vi "testUDPReciever.vi"() -> ()   [LabVIEW 2012]
panel:
  out "word 3":u8[](array[numeric]) format="%02x"
  out "word 2":u8[](array[numeric]) format="%02x"
  out "word 1":u8[](array[numeric]) format="%02x"
  out "word 0":u8[](array[numeric]) format="%02x"
  out "i":i32
  out "Found Header":bool
  out "MultiDimHeader":bool[][](array[boolean])
  out "NumBins":u32
  out "Cnts/Bin":u32
  out "Prof/Hist":u32
  out "Sync":u32
  out "Channel":u32
  out "rTime":u32
  out "frameCntr":u32
  out "subarray":bool[](array[boolean])
  out "channel 11":u32[](graph)
  out "in 11":bool
  out "channel 10":u32[](graph)
  out "in 10":bool
  out "channel 9":u32[](graph)
  out "in 9":bool
  out "channel 8":u32[](graph)
  out "in 8":bool
  out "channel 7":u32[](graph)
  out "in 7":bool
  out "channel 6":u32[](graph)
  out "in 6":bool
  out "channel 5":u32[](graph)
  out "in 5":bool
  out "channel 4":u32[](graph)
  out "in 4":bool
  out "channel 3":u32[](graph)
  out "in 3":bool
  out "channel 2":u32[](graph)
  out "in 2":bool
  out "channel 1":u32[](graph)
  out "in 1":bool
  out "channel 0":u32[](graph)
  out "in 0":bool
  out "appended array 2":string[](array[string])
  out "channel":u32
  out "appended array":bool[][](array[boolean])
  out "Found Header 2":bool
  out "word 7":u8[](array[numeric]) format="%02x"
  out "word 6":u8[](array[numeric]) format="%02x"
  out "word 5":u8[](array[numeric]) format="%02x"
  out "word 4":u8[](array[numeric]) format="%02x"
  out "Raw Data Out":string
  out "error post-check":errorcluster
  out "End Reciever Error":errorcluster
  in  "stop reciever":bool
  out "port":u16
  out "error out post-read":errorcluster
  out "error out pre-read":errorcluster
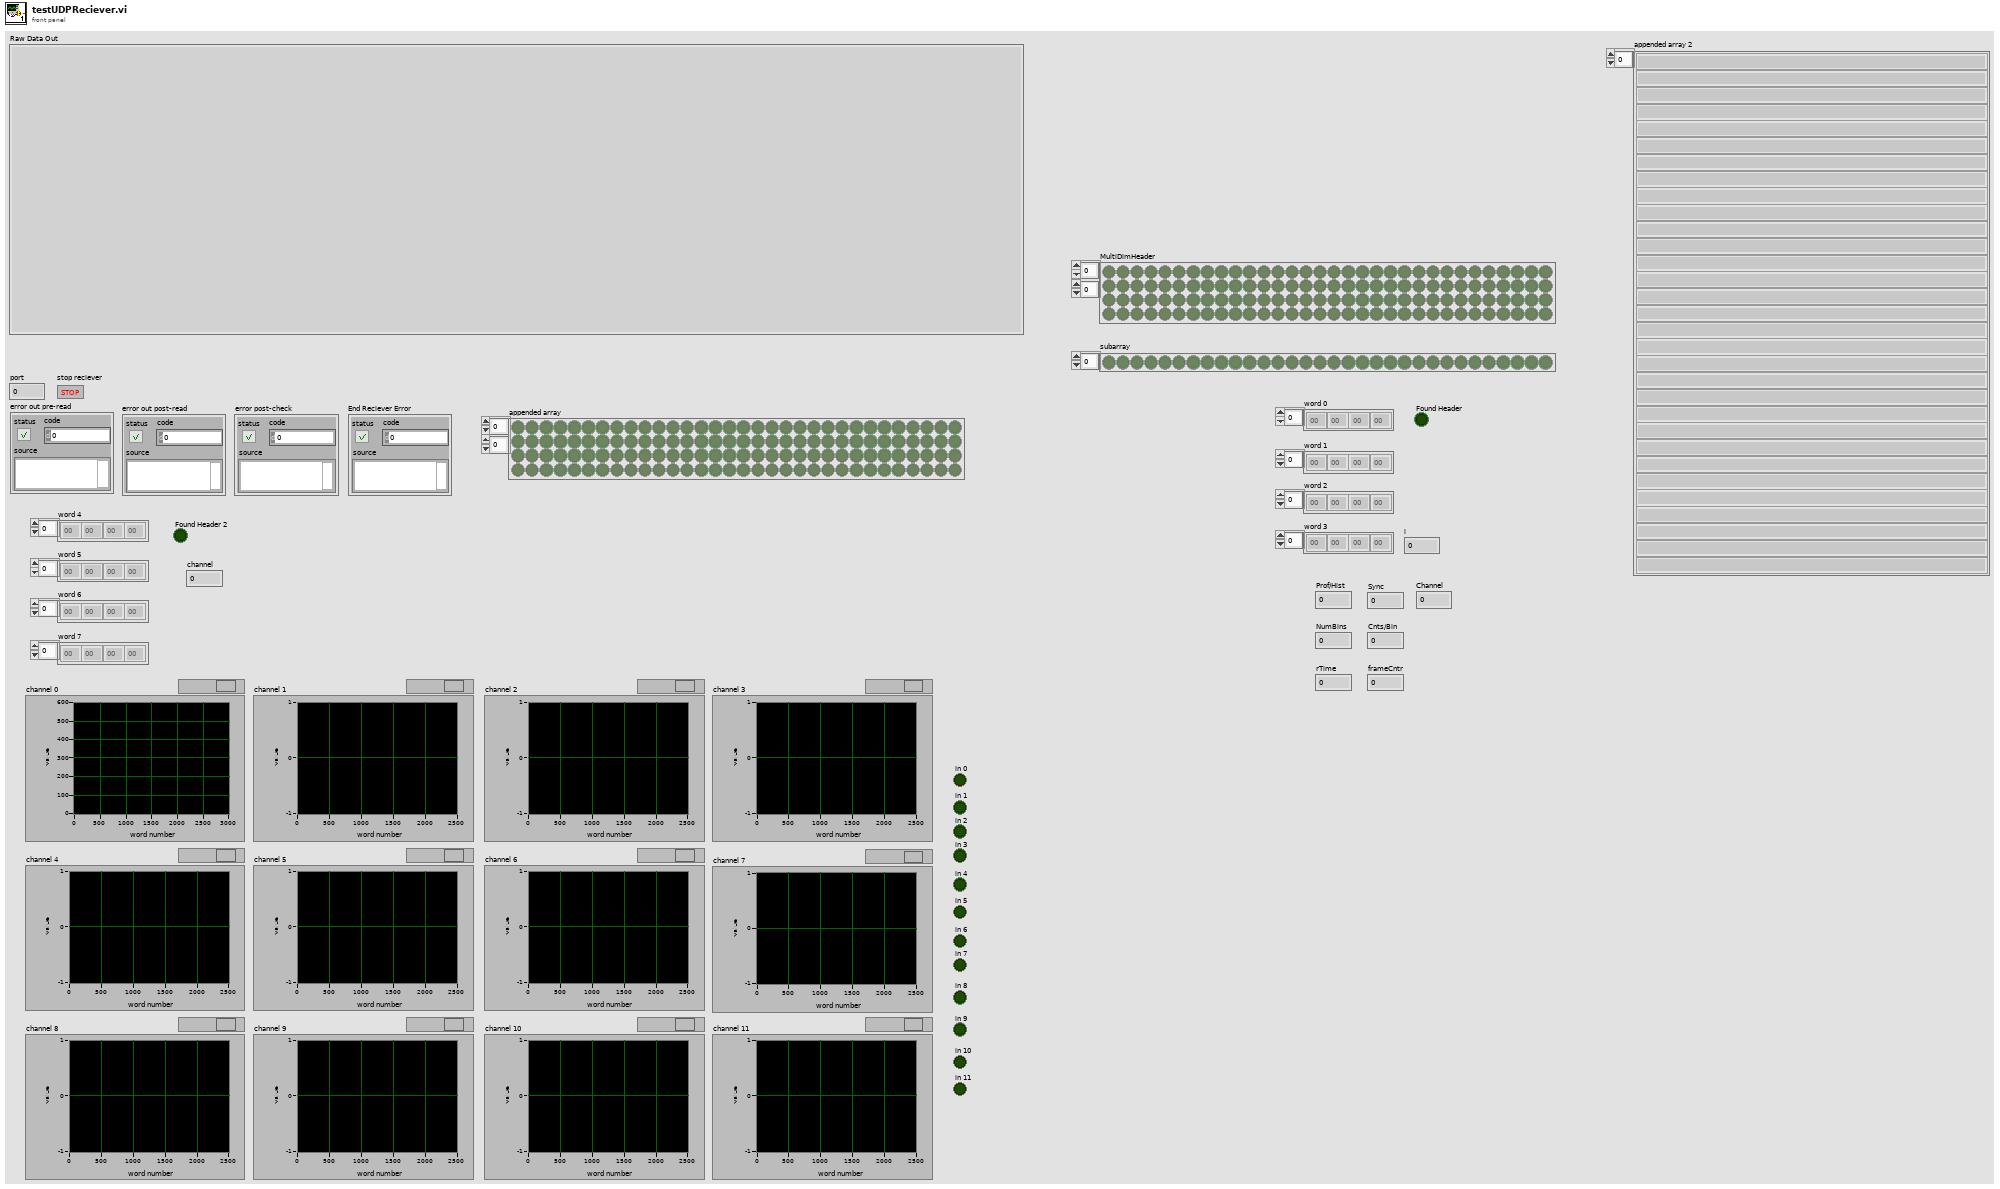
[diagram p1: front panel]
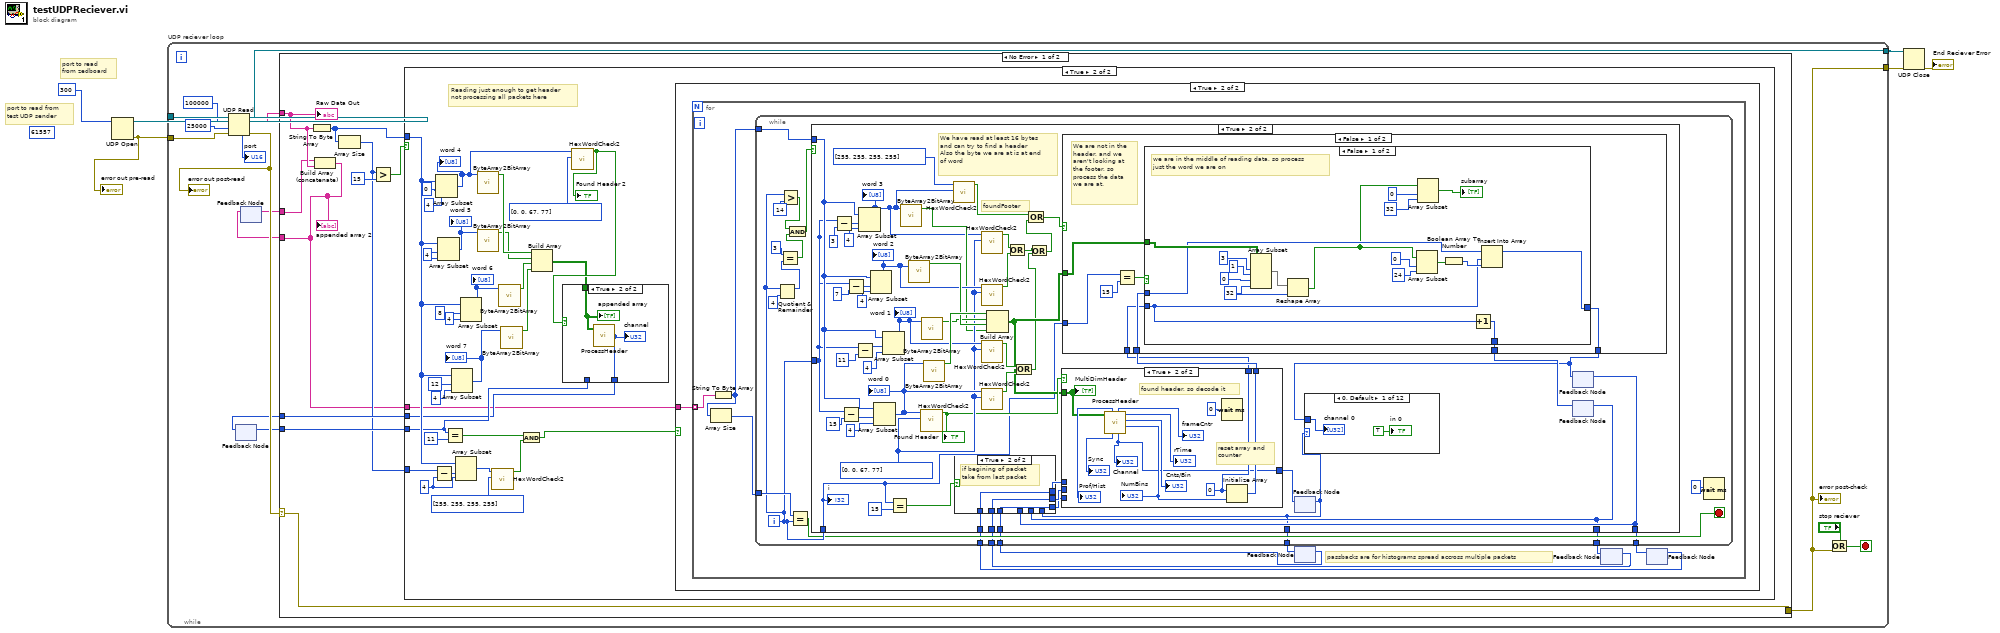
[diagram p0: block diagram]
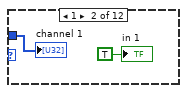
[diagram p5: hidden frame]
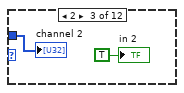
[diagram p6: hidden frame]
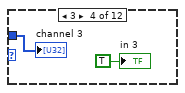
[diagram p7: hidden frame]
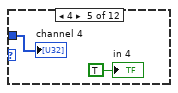
[diagram p8: hidden frame]
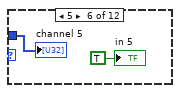
[diagram p9: hidden frame]
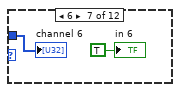
[diagram p10: hidden frame]
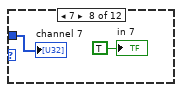
[diagram p11: hidden frame]
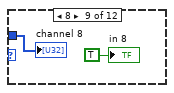
[diagram p12: hidden frame]
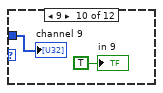
[diagram p13: hidden frame]
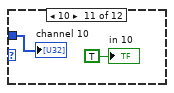
[diagram p14: hidden frame]
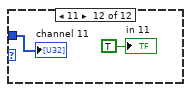
[diagram p15: hidden frame]
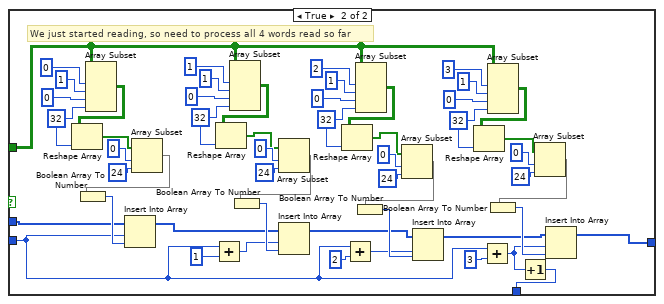
[diagram p17: hidden frame]
diagram:
  (unwired) u16 61557 ("port")
  # "port to read \nfrom zedboard"
  # "port to read from \ntest UDP sender"
  n1 = UDP Open(11:u16 300 ("port")) -> (port=w5:refnum<k16>, 0:w2:errorcluster)  [unwired: 4 in, 1 out]
  "error out pre-read" <- w2
  n2 = while "UDP reciever loop" {
    tunnel: [w21] -> w6
    tunnel: w5 -> [w20]
    tunnel: [w12] -> w4
    tunnel: w2 -> [w17]
    stop <- w19 stop-if-true
    n3 = UDP Read(connection ID=w20, max size (548)=100000, timeout ms (25000)=25000, 8:w17) -> (data out=w14:string, error out=w16:errorcluster, 3:w21:refnum<k16>, 4:→"port":u16)  [unwired: 1 out]
    "error out post-read" <- w16
    n4 = feedback #1() -> (w7:u32)  [unwired: 1 in]
    n5 = feedback #2() -> (w9:string[])  [unwired: 1 in]
    n6 = case shown="No Error" w16 {
      selector: w16 -> [w31 w278]
      tunnel: w14 -> [w30 _]
      tunnel: [w31 w278] -> w12
      tunnel: [w23 w277] -> w10
      tunnel: w9 -> [w29 w277]
      tunnel: [w26 w276] -> w8
      tunnel: w7 -> [w25 w276]
      frame No Error {
        n7 = String To Byte Array(string=w30) -> (unsigned byte array=w22:u8[])
        n8 = Build Array (concatenate)(w29, w30) -> (w23:string[])
        "appended array 2" <- w23
        n9 = Array Size(array=w22) -> (size(s)=w24:i32)
        n10 = Greater?(x=w24, y=15) -> (0:w28:bool)
        n11 = case shown="True" w28 {
          tunnel: w22 -> [_ w40]
          tunnel: [w32 w34] -> w26
          tunnel: w25 -> [w32 w35]
          tunnel: w24 -> [_ w37]
          tunnel: w23 -> [_ w33]
          frame False {
          }
          frame True {
            w39 = 4 ("length")
            w58 = 4 ("length")
            # "Reading just enough to get header\nnot processing all packets here"
            n12 = Subtract(x=w37, y=w39) -> (x-y=w38:i32)
            n13 = Array Subset(array=w40, index=0, length=4) -> (w47:u8[])
            "word 4" <- w47
            n14 = Array Subset(array=w40, index=w58, length=w58) -> (w63:u8[])
            "word 5" <- w63
            n15 = Equal?(x=w35, y=u32 11) -> (x = y?=w42:bool)
            n16 = Array Subset(array=w40, index=12, length=4) -> (w45:u8[])
            "word 7" <- w45
            n17 = Array Subset(array=w40, index=w38, length=w39) -> (w36:u8[])
            n18 = Array Subset(array=w40, index=8, length=4) -> (w62:u8[])
            "word 6" <- w62
            n19 = call "ByteArray2BitArray.vi"("array"=w47) -> ("Array"=w53:bool[])  [unwired: 10 in]
            n20 = call "ByteArray2BitArray.vi"("array"=w63) -> ("Array"=w52:bool[])  [unwired: 10 in]
            n21 = call "HexWordCheck2.vi"("array"=u8[] [255, 255, 255, 255], "Input Array"=w36) -> ("Boolean"=w41:bool)  [unwired: 9 in]
            n22 = call "ByteArray2BitArray.vi"("array"=w62) -> ("Array"=w50:bool[])  [unwired: 10 in]
            n23 = call "ByteArray2BitArray.vi"("array"=w45) -> ("Array"=w51:bool[])  [unwired: 10 in]
            n24 = And(x=w42, y=w41) -> (x .and. y?=w44:bool)
            n25 = Build Array(w53, w52, w50, w51) -> (w48:bool[][])
            n26 = call "HexWordCheck2.vi"("array"=u8[] [0, 0, 67, 77], "Input Array"=w47) -> ("Boolean"=w49:bool)  [unwired: 9 in]
            "Found Header 2" <- w49
            n27 = case shown="True" w49 {
              tunnel: w48 -> [_ w275]
              tunnel: [w273 w274] -> w34
              tunnel: w35 -> [w273 _]
              frame False {
              }
              frame True {
                n28 = call "ProcessHeader.vi"("Array"=w275) -> ("Numeric 4"=w274:u32)  [unwired: 4 in, 6 out]
                "channel" <- w274
                "appended array" <- w275
              }
            }
            n29 = case shown="True" w44 {
              tunnel: w33 -> [_ w64]
              frame False {
              }
              frame True {
                n30 = for {
                  tunnel: w64 -> [w73] mode=indexing
                  # "passbacks are for histograms spread accross multiple packets"
                  n31 = String To Byte Array(string=w73) -> (unsigned byte array=w65:u8[])
                  n32 = Array Size(array=w65) -> (size(s)=w66:i32)
                  n33 = feedback #3() -> (w67:u32)  [unwired: 1 in]
                  n34 = feedback #4() -> (w69:u32)  [unwired: 1 in]
                  n35 = feedback #5() -> (w70:u32[])  [unwired: 1 in]
                  n36 = while {
                    tunnel: w65 -> [w88]
                    tunnel: w66 -> [w91]
                    tunnel: [w79] -> w72
                    tunnel: [w78] -> w71
                    tunnel: w70 -> [w77]
                    tunnel: w69 -> [w76]
                    tunnel: [w75] -> w68
                    tunnel: w67 -> [w74]
                    i -> [w87]
                    stop <- w80 stop-if-true
                    n37 = Quotient & Remainder(x=w87, y=4) -> (x-y*floor(x/y)=w85:i32)  [unwired: 1 out]
                    n38 = Equal?(x=3, y=w85) -> (x = y?=w81:bool)
                    n39 = Greater?(x=w87, y=14 ("x")) -> (0:w83:bool)
                    n40 = And(x=w83, y=w81) -> (x .and. y?=w82:bool)
                    n41 = Equal?(x=w91, y=w87) -> (x = y?=w80:bool)
                    n42 = case shown="True" w82 {
                      tunnel: w88 -> [_ w131]
                      tunnel: w87 -> [_ w130]
                      tunnel: w87 -> [_ w105]
                      tunnel: [w94 w108] -> w79
                      tunnel: [w93 w101] -> w78
                      tunnel: w77 -> [w94 w110]
                      tunnel: w76 -> [w93 w109]
                      tunnel: [w92 w96] -> w75
                      tunnel: w74 -> [w92 w99]
                      frame False {
                      }
                      frame True {
                        w120 = u8[] [0, 0, 67, 77] ("array")
                        # "foundFooter"
                        # "We have read at least 16 bytes \nand can try to find a header\nAlso the byte we are at is at end \nof word"
                        n43 = Subtract(x=w130, y=3) -> (x-y=w146:i32)
                        n44 = Subtract(x=w130, y=15) -> (x-y=w140:i32)
                        n45 = Subtract(x=w130, y=7) -> (x-y=w144:i32)
                        n46 = Subtract(x=w130, y=11) -> (x-y=w142:i32)
                        n47 = Array Subset(array=w131, index=w146, length=4) -> (w115:u8[])
                        "word 3" <- w115
                        n48 = Array Subset(array=w131, index=w144, length=4) -> (w129:u8[])
                        "word 2" <- w129
                        n49 = Array Subset(array=w131, index=w140, length=4) -> (w122:u8[])
                        "word 0" <- w122
                        n50 = Array Subset(array=w131, index=w142, length=4) -> (w128:u8[])
                        "word 1" <- w128
                        n51 = Equal?(x=w105, y=15) -> (x = y?=w103:bool)
                        n52 = call "ByteArray2BitArray.vi"("array"=w115) -> ("Array"=w117:bool[])  [unwired: 10 in]
                        n53 = call "ByteArray2BitArray.vi"("array"=w129) -> ("Array"=w133:bool[])  [unwired: 10 in]
                        n54 = call "HexWordCheck2.vi"("array"=w120, "Input Array"=w122) -> ("Boolean"=w119:bool)  [unwired: 9 in]
                        "Found Header" <- w119
                        n55 = call "ByteArray2BitArray.vi"("array"=w128) -> ("Array"=w132:bool[])  [unwired: 10 in]
                        n56 = call "ByteArray2BitArray.vi"("array"=w122) -> ("Array"=w134:bool[])  [unwired: 10 in]
                        n57 = call "HexWordCheck2.vi"("array"=w115, "Input Array"=u8[] [255, 255, 255, 255] ("array")) -> ("Boolean"=w100:bool)  [unwired: 9 in]
                        n58 = call "HexWordCheck2.vi"("array"=w120, "Input Array"=w115) -> ("Boolean"=w125:bool)  [unwired: 9 in]
                        n59 = call "HexWordCheck2.vi"("array"=w120, "Input Array"=w129) -> ("Boolean"=w124:bool)  [unwired: 9 in]
                        n60 = call "HexWordCheck2.vi"("array"=w120, "Input Array"=w128) -> ("Boolean"=w126:bool)  [unwired: 9 in]
                        n61 = call "HexWordCheck2.vi"("array"=w120, "Input Array"=w122) -> ("Boolean"=w127:bool)  [unwired: 9 in]
                        n62 = Build Array(w134, w132, w133, w117) -> (w118:bool[][])
                        n63 = Or(x=w125, y=w124) -> (x .or. y?=w123:bool)
                        n64 = Or(x=w126, y=w127) -> (x .or. y?=w111:bool)
                        n65 = Or(x=w123, y=w111) -> (x .or. y?=w114:bool)
                        n66 = Or(x=w100, y=w114) -> (x .or. y?=w113:bool)
                        n67 = feedback #6() -> (w96:u32)  [unwired: 1 in]
                        n68 = feedback #7() -> (w108:u32[])  [unwired: 1 in]
                        n69 = feedback #8() -> (w101:u32)  [unwired: 1 in]
                        n70 = case shown="True" w103 {
                          tunnel: w110 -> [_ w176]
                          tunnel: w109 -> [_ w175]
                          tunnel: w101 -> [w172 _]
                          tunnel: w108 -> [w173 _]
                          tunnel: [w172 w175] -> w107
                          tunnel: [w173 w176] -> w106
                          tunnel: w99 -> [_ w174]
                          tunnel: [w171 w174] -> w98
                          tunnel: w96 -> [w171 _]
                          frame False {
                            # "if middle of packet\ntake from this loop"
                          }
                          frame True {
                            # "if begining of packet\ntake from last packet"
                          }
                        }
                        n71 = case shown="True" w119 {
                          tunnel: w118 -> [_ w268]
                          tunnel: [w260 w265] -> w121
                          tunnel: [w261 w263] -> w112
                          tunnel: w107 -> [w261 _]
                          tunnel: w106 -> [w260 _]
                          tunnel: [w259 w262] -> w97
                          tunnel: w98 -> [w259 _]
                          frame False {
                            # "didn't find header so keep info from \nlast itteration of loop"
                          }
                          frame True {
                            w263 = u32 0 ("element")
                            # "reset array and \ncounter"
                            # "found header, so decode it"
                            n72 = call "ProcessHeader.vi"("Array"=w268) -> ("Numeric"=w264:u32, "Numeric 7"=→"Cnts/Bin":u32, "Numeric 3"=→"rTime":u32, "Numeric 4"=w262:u32, "Numeric 2"=→"frameCntr":u32, "Numeric 5"=→"Sync":u32, "Numeric 6"=→"Prof/Hist":u32)  [unwired: 4 in]
                            "NumBins" <- w264
                            "Channel" <- w262
                            n73 = Wait (ms)(milliseconds to wait=u32 0) -> ()  [unwired: 1 out]
                            n74 = Initialize Array(w263, w264) -> (w265:u32[])
                            "MultiDimHeader" <- w268
                          }
                        }
                        n75 = case shown="False" w113 {
                          tunnel: w105 -> [w179 _]
                          tunnel: w121 -> [w180 w258]
                          tunnel: [w181 w258] -> w95
                          tunnel: w118 -> [w182 _]
                          tunnel: w112 -> [w178 w257]
                          tunnel: [w177 w257] -> w102
                          frame False {
                            # "We are not in the \nheader, and we \naren't looking at \nthe footer, so \nprocess the data \nwe are at."
                            n76 = Equal?(x=w179, y=15) -> (x = y?=w183:bool)
                            n77 = case shown="False" w183 {
                              tunnel: w182 -> [w193 w236]
                              tunnel: [w191 w211] -> w181
                              tunnel: w180 -> [w192 w230]
                              tunnel: w178 -> [w189 w208]
                              tunnel: [w190 w204] -> w177
                              frame False {
                                w202 = 32 ("length")
                                # "we are in the middle of reading data, so process \njust the word we are on"
                                n78 = Array Subset(array=w193, index (row)=3 ("index"), length (row)=1 ("length"), index (col)=0 ("index"), length (col)=w202) -> (w201:bool[][])
                                n79 = Reshape Array(w201, w202) -> (w188:bool[])
                                n80 = Array Subset(array=w188, index=0, length=24) -> (w194:bool[])
                                n81 = Array Subset(array=w188, index=0, length=32) -> (→"subarray":bool[])
                                n82 = Boolean Array To Number(Boolean array=w194) -> (number=w197:u32)
                                n83 = Increment(x=w189) -> (x+1=w190:u32)
                                n84 = Insert Into Array(array=w192, index=w189, new element=w197) -> (w191:u32[])
                              }
                              frame True {
                                w238 = 32 ("length")
                                w243 = 32 ("length")
                                w248 = 32 ("length")
                                w253 = 32 ("length")
                                # "We just started reading, so need to process all 4 words read so far"
                                n85 = Array Subset(array=w236, index (row)=0 ("index"), length (row)=1 ("length"), index (col)=0 ("index"), length (col)=w253) -> (w252:bool[][])
                                n86 = Reshape Array(w252, w253) -> (w231:bool[])
                                n87 = Array Subset(array=w231, index=0, length=24) -> (w235:bool[])
                                n88 = Boolean Array To Number(Boolean array=w235) -> (number=w232:u32)
                                n89 = Insert Into Array(array=w230, index=w208, new element=w232) -> (w224:u32[])
                                n90 = Add(x=w208, y=u32 1) -> (x+y=w209:u32)
                                n91 = Array Subset(array=w236, index (row)=1 ("index"), length (row)=1 ("length"), index (col)=0 ("index"), length (col)=w248) -> (w247:bool[][])
                                n92 = Reshape Array(w247, w248) -> (w227:bool[])
                                n93 = Array Subset(array=w227, index=0, length=24) -> (w225:bool[])
                                n94 = Boolean Array To Number(Boolean array=w225) -> (number=w226:u32)
                                n95 = Insert Into Array(array=w224, index=w209, new element=w226) -> (w218:u32[])
                                n96 = Add(x=w208, y=u32 2) -> (x+y=w210:u32)
                                n97 = Array Subset(array=w236, index (row)=2 ("index"), length (row)=1 ("length"), index (col)=0 ("index"), length (col)=w243) -> (w242:bool[][])
                                n98 = Reshape Array(w242, w243) -> (w220:bool[])
                                n99 = Array Subset(array=w220, index=0, length=24) -> (w219:bool[])
                                n100 = Boolean Array To Number(Boolean array=w219) -> (number=w221:u32)
                                n101 = Insert Into Array(array=w218, index=w210, new element=w221) -> (w212:u32[])
                                n102 = Add(x=w208, y=u32 3) -> (x+y=w203:u32)
                                n103 = Array Subset(array=w236, index (row)=3 ("index"), length (row)=1 ("length"), index (col)=0 ("index"), length (col)=w238) -> (w237:bool[][])
                                n104 = Reshape Array(w237, w238) -> (w214:bool[])
                                n105 = Increment(x=w203) -> (x+1=w204:u32)
                                n106 = Array Subset(array=w214, index=0, length=24) -> (w213:bool[])
                                n107 = Boolean Array To Number(Boolean array=w213) -> (number=w215:u32)
                                n108 = Insert Into Array(array=w212, index=w203, new element=w215) -> (w211:u32[])
                              }
                            }
                          }
                          frame True {
                          }
                        }
                        n109 = feedback-in #6(w97) -> ()
                        n110 = case shown="0, Default" w96 {
                          tunnel: w95 -> [w148 w150 w152 w154 w156 w158 w160 w162 w164 w166 w168 w170]
                          frame 0, Default {
                            "channel 0" <- w148
                            "in 0" <- TRUE ("in 11")
                          }
                          frame 1 {
                            "channel 1" <- w150
                            "in 1" <- TRUE ("in 11")
                          }
                          frame 2 {
                            "channel 2" <- w152
                            "in 2" <- TRUE ("in 11")
                          }
                          frame 3 {
                            "channel 3" <- w154
                            "in 3" <- TRUE ("in 11")
                          }
                          frame 4 {
                            "channel 4" <- w156
                            "in 4" <- TRUE ("in 11")
                          }
                          frame 5 {
                            "channel 5" <- w158
                            "in 5" <- TRUE ("in 11")
                          }
                          frame 6 {
                            "channel 6" <- w160
                            "in 6" <- TRUE ("in 11")
                          }
                          frame 7 {
                            "channel 7" <- w162
                            "in 7" <- TRUE ("in 11")
                          }
                          frame 8 {
                            "channel 8" <- w164
                            "in 8" <- TRUE ("in 11")
                          }
                          frame 9 {
                            "channel 9" <- w166
                            "in 9" <- TRUE ("in 11")
                          }
                          frame 10 {
                            "channel 10" <- w168
                            "in 10" <- TRUE ("in 11")
                          }
                          frame 11 {
                            "channel 11" <- w170
                            "in 11" <- TRUE ("in 11")
                          }
                        }
                        n111 = feedback-in #7(w95) -> ()
                        n112 = feedback-in #8(w102) -> ()
                        "i" <- w105
                      }
                    }
                    n113 = Wait (ms)(milliseconds to wait=u32 0) -> ()  [unwired: 1 out]
                  }
                  n114 = feedback-in #3(w68) -> ()
                  n115 = feedback-in #4(w71) -> ()
                  n116 = feedback-in #5(w72) -> ()
                }
              }
            }
          }
        }
        "Raw Data Out" <- w30
      }
      frame Error {
      }
    }
    "error post-check" <- w12
    n117 = feedback-in #1(w8) -> ()
    n118 = feedback-in #2(w10) -> ()
    n119 = Or(x="stop reciever", y=w12) -> (x .or. y?=w19:bool)
  }
  n120 = UDP Close(connection ID=w6, 8:w4) -> (error out=→"End Reciever Error":errorcluster)  [unwired: 1 out]
